vi "Exponential Fit Coefficients (LS).vi"(0 "Y":dbl[](array[numeric]) format="%0.2f", 5 "X":dbl[](array[numeric]) format="%0.2f", 7 "Weight":dbl[](array[numeric]), 9 "tolerance":dbl=0.0001 format="%#_3g", 11 "Initial Coefficients":dbl[](array[numeric]), 12 "algorithm":u16(ring) items=["Semi-Log", "Iterative"]) -> (4 "amplitude":dbl format="%0.2f", 6 "damping":dbl format="%0.2f", 15 "error":i32)   [LabVIEW 2017, in "NI_AALPro.lvlib"]
uses:
  NI_AALPro.lvlib
  lvanlys.dll
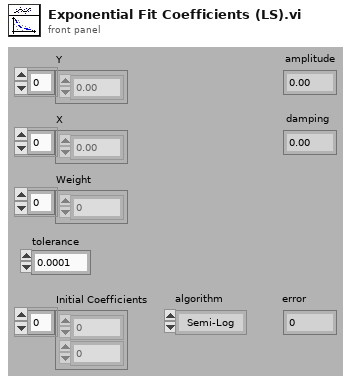
[diagram p1: front panel]
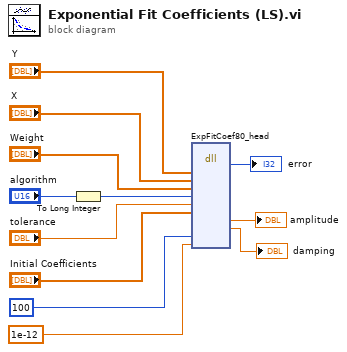
[diagram p0: block diagram]
diagram:
  n1 = To Long Integer(number="algorithm") -> (32bit integer=w6:i32)
  n2 = dll-call lib="C:/Program Files/National Instruments/LabVIEW 2017/resource/lvanlys.*" fn="ExpFitCoef80_head"("yH"="Y", "xH"="X", "weightH"="Weight", "algorithm"=w6, "tol"="tolerance", "initialCoefH"="Initial Coefficients", "maxIter"=100, "absTol"=1e-12) -> (→"error":i32, "amplitude"=→"amplitude":dbl, "damping"=→"damping":dbl)  [unwired: 13 in, 2 out]
